vi "Get product of adjacent numbers-diagonal.vi"(8 "error in (no error)":errorcluster, 9 "Diagonal direction":T1, 10 "How many adjacent numbers? (dflt=4)":i32=4, 11 "2D array":i32[][](array[numeric])=[[8, 2, 22, 97, 38, 15, 0, 40, 0, 75, 4, 5, 7, 78, 52, 12, 50, 77, 91, 8], [49, 49, 99, 40, 17, 81, 18, 57, 60, 87, 17, 40, 98, 43, 69, 48, 4, 56, 62, 0], [81, 49, 31, 73, 55, 79, 14, 29, 93, 71, 40, 67, 53, 88, 30, 3, 49, 13, 36, 65], [52, 70, 95, 23, 4, 60, 11, 42, 69, 24, 68, 56, 1, 32, 56, 71, 37, 2, 36, 91], [22, 31, 16, 71, 51, 67, 63, 89, 41, 92, 36, 54, 22, 40, 40, 28, 66, 33, 13, 80], [24, 47, 32, 60, 99, 3, 45, 2, 44, 75, 33, 53, 78, 36, 84, 20, 35, 17, 12, 50], [32, 98, 81, 28, 64, 23, 67, 10, 26, 38, 40, 67, 59, 54, 70, 66, 18, 38, 64, 70], [67, 26, 20, 68, 2, 62, 12, 20, 95, 63, 94, 39, 63, 8, 40, 91, 66, 49, 94, 21], [24, 55, 58, 5, 66, 73, 99, 26, 97, 17, 78, 78, 96, 83, 14, 88, 34, 89, 63, 72], [21, 36, 23, 9, 75, 0, 76, 44, 20, 45, 35, 14, 0, 61, 33, 97, 34, 31, 33, 95], [78, 17, 53, 28, 22, 75, 31, 67, 15, 94, 3, 80, 4, 62, 16, 14, 9, 53, 56, 92], [16, 39, 5, 42, 96, 35, 31, 47, 55, 58, 88, 24, 0, 17, 54, 24, 36, 29, 85, 57], [86, 56, 0, 48, 35, 71, 89, 7, 5, 44, 44, 37, 44, 60, 21, 58, 51, 54, 17, 58], [19, 80, 81, 68, 5, 94, 47, 69, 28, 73, 92, 13, 86, 52, 17, 77, 4, 89, 55, 40], [4, 52, 8, 83, 97, 35, 99, 16, 7, 97, 57, 32, 16, 26, 26, 79, 33, 27, 98, 66], [88, 36, 68, 87, 57, 62, 20, 72, 3, 46, 33, 67, 46, 55, 12, 32, 63, 93, 53, 69], [4, 42, 16, 73, 38, 25, 39, 11, 24, 94, 72, 18, 8, 46, 29, 32, 40, 62, 76, 36], [20, 69, 36, 41, 72, 30, 23, 88, 34, 62, 99, 69, 82, 67, 59, 85, 74, 4, 36, 16], [20, 73, 35, 29, 78, 31, 90, 1, 74, 31, 49, 71, 48, 86, 81, 16, 23, 57, 5, 54], [1, 70, 54, 71, 83, 51, 54, 69, 16, 92, 33, 48, 61, 43, 52, 1, 89, 19, 67, 48]]) -> (0 "error out":errorcluster, 3 "Highest product-diagonal direction":u64)   [LabVIEW 2021, in "Project Euler.lvlib"]
uses:
  Project Euler.lvlib
  Utilities/Numeric Utilities/diagonal direction.ctl
  Utilities/Numeric Utilities/Numeric Utilities.lvlib
panel:
  out "no. of products":i32
  out "All products":u64[](array[numeric])
  out "no. of columns":i32
  out "no. of rows":i32
  # "Development\ncontrols/indicators useful for development and testing, but which are not outputs of the VI"
  # "Input\nInputs to the VI"
  # "Output\nOutputs of the VI"
  # "Description\n\nBlank VI with error handling case. \n\nSummarize the use of this VI in this space."
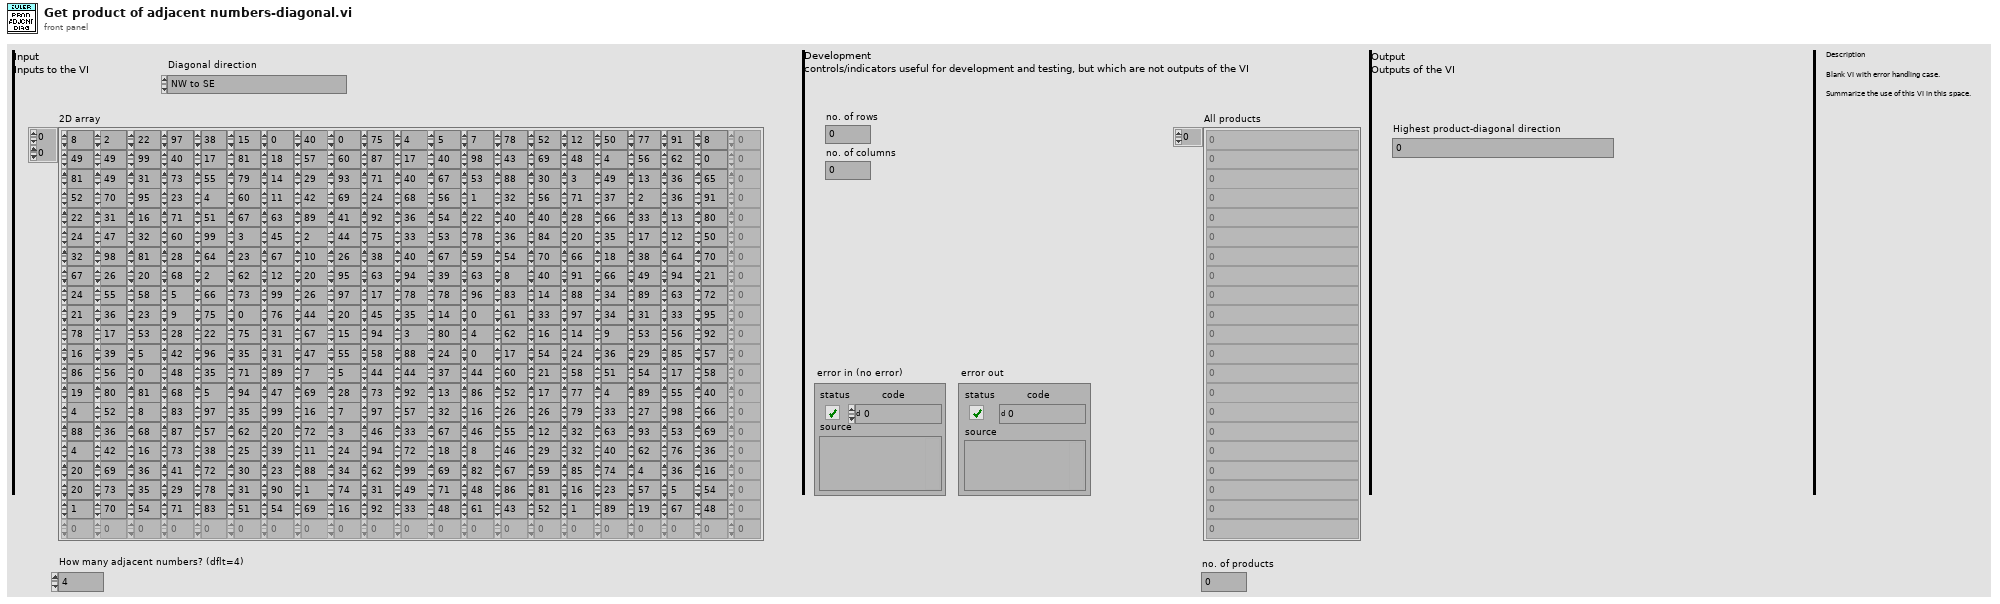
[diagram p1: front panel]
types:
  T1 = typedef "Numeric Utilities.lvlib/diagonal direction.ctl" = enum16{"NW to SE", "SE to NW", "NE to SW", "SW to NE"}
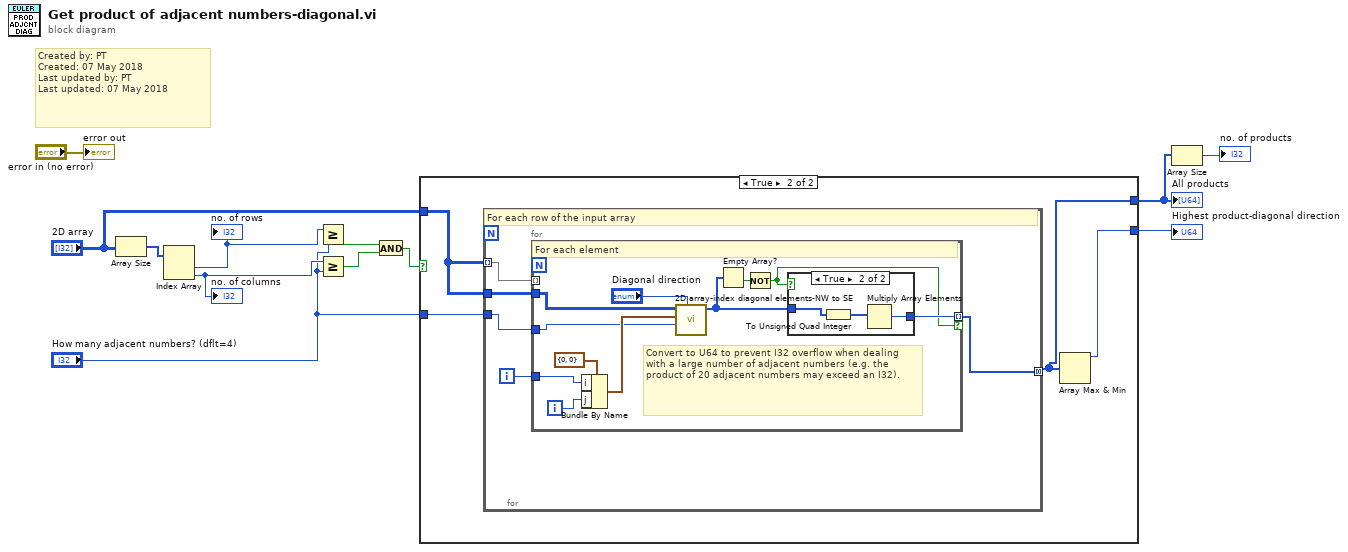
[diagram p0: block diagram]
diagram:
  # "Created by: PT\nCreated: 07 May 2018\nLast updated by: PT\nLast updated: 07 May 2018"
  n1 = Array Size(array="2D array") -> (size(s)=w10:i32[])
  n2 = Index Array(array=w10) -> (element #1=w5:i32, element #2=w6:i32)  [unwired: 2 in]
  "no. of rows" <- w5
  "no. of columns" <- w6
  n3 = Greater Or Equal?(x=w5, y="How many adjacent numbers? (dflt=4)") -> (x >= y?=w3:bool)
  n4 = Greater Or Equal?(x=w6, y="How many adjacent numbers? (dflt=4)") -> (x >= y?=w2:bool)
  n5 = And(x=w3, y=w2) -> (x .and. y?=w1:bool)
  n6 = case shown="True" w1 {
    tunnel: [_ w15] -> w11
    tunnel: "2D array" -> [_ w13]
    tunnel: "How many adjacent numbers? (dflt=4)" -> [_ w16]
    tunnel: [_ w14] -> w8
    frame False {
    }
    frame True {
      n7 = for {
        tunnel: w13 -> [w21] mode=indexing
        tunnel: w16 -> [w20]
        tunnel: [w17] -> w14 mode=concatenating
        tunnel: w13 -> [w19]
        i -> [w18]
        # "For each row of the input array"
        n8 = for {
          tunnel: w21 -> [_] mode=indexing
          tunnel: w20 -> [w27]
          tunnel: w19 -> [w32]
          tunnel: w18 -> [w31]
          tunnel: [w25] -> w17 mode=indexing if=w22
          i -> [w30]
          # "Convert to U64 to prevent I32 overflow when dealing with a large number of adjacent numbers (e.g. the product of 20 adjacent numbers may exceed an I32)."
          # "For each element"
          n9 = Bundle By Name(cluster=cluster{"i":u32, "j":u32} {"i"=0, "j"=0} ("index of first element"), "i"=w31, "j"=w30) -> (w28:cluster{"i":u32, "j":u32})
          n10 = call "2D array-index diagonal elements-NW to SE.vi"("Diagonal direction"="Diagonal direction", "no. of elements (dflt=4)"=w27, "index of first element"=w28, "2D array in"=w32) -> ("Diagonal elements out"=w24:i32[])  [unwired: 6 in, 1 out]
          n11 = Empty Array?(array=w24) -> (empty?=w23:bool)
          n12 = Not(x=w23) -> (.not. x?=w22:bool)
          n13 = case shown="True" w22 {
            tunnel: w24 -> [_ w34]
            tunnel: [_ w33] -> w25
            frame False {
            }
            frame True {
              n14 = To Unsigned Quad Integer(1:w34) -> (0:w35:u64[])
              n15 = Multiply Array Elements(1:w35) -> (0:w33:u64)
            }
          }
        }
      }
      n16 = Array Max & Min(array=w14) -> (max value=w15:u64)  [unwired: 3 out]
    }
  }
  "Highest product-diagonal direction" <- w11
  "All products" <- w8
  n17 = Array Size(array=w8) -> (size(s)=→"no. of products":i32)
  "error out" <- "error in (no error)"
